vi "ACTION.vi"(8 "error in (no error)":errorcluster, 9 "STEP State":T1, 10 "CORE":refnum<queue>, 11 "Measurement wRelev in":refnum<class "Measurement wRelev.lvclass">) -> (0 "error out":errorcluster, 3 "Measurement wRelev out":refnum<class "Measurement wRelev.lvclass">)   [LabVIEW 2014, in "SeqLoop.lvlib" / "STEP Classes.lvlib" / "Measurement wRelev.lvclass"]
uses:
  Measurement wRelev.lvclass
  TypeDefs/STEP State.ctl
  APIs/Message Queue/Message Cluster.ctl
  Measurement wRelev.lvclass/Measurement wRelev.ctl
  APIs/Message Queue/Enqueue Message (Array).vi
  APIs/Message Queue/Enqueue Message (Single).vi
  APIs/Message Queue/WINFAS 2 Message Queue.lvlib
  SeqLoop.lvlib
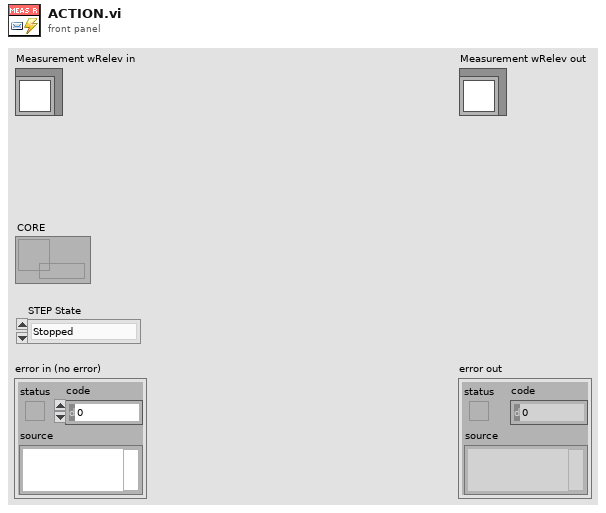
[diagram p1: front panel]
types:
  T1 = typedef "SeqLoop.lvlib/STEP State.ctl" = enum16{"Stopped", "First Call", "Idle...", "Advance OK", "Alarm", "Output Security", "Error"}
  T2 = cluster{"HWSync 1":bool, "HWSync 2":bool, "HWSync 3":bool, "HWSync 4":bool, "HWSync 5":bool}
  T3 = cluster{"HWAsync 1":string, "HWAsync 2":string, "HWAsync 3":string, "HWAsync 4":string, "HWAsync 5":string, "HWAsync 6":string, "HWAsync 7":string, "HWAsync 8":string, "HWAsync 9":string, "HWAsync 10":string}
  T4 = cluster{"format string":string, "Measurement Index":i32[]}
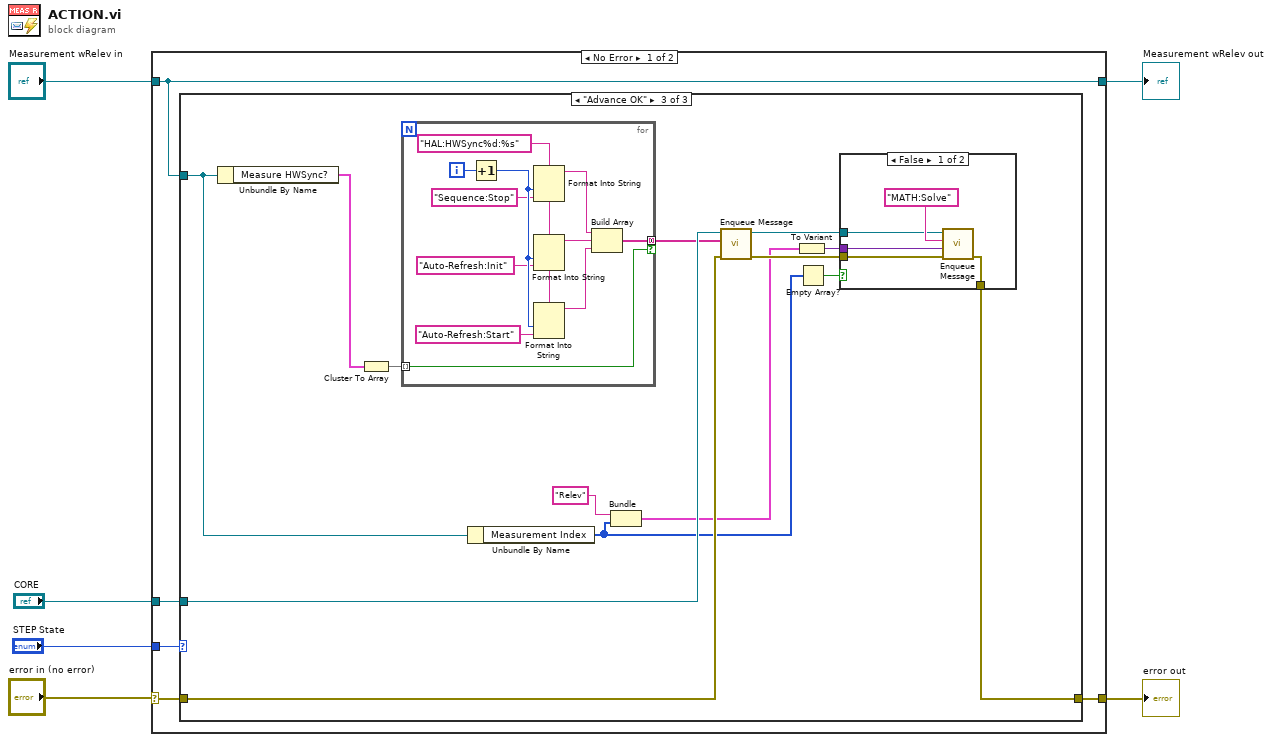
[diagram p0: block diagram]
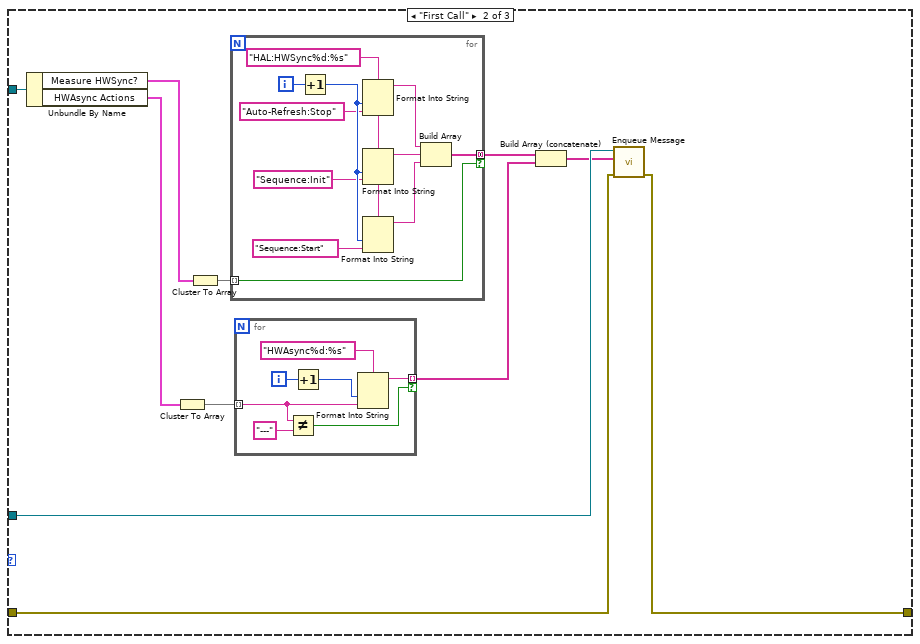
[diagram p3: hidden frame]
diagram:
  n1 = case shown="No Error" "error in (no error)" {
    selector: "error in (no error)" -> [w8 w74]
    tunnel: [w7 w74] -> w3
    tunnel: [w11 w73] -> w5
    tunnel: "Measurement wRelev in" -> [w11 w73]
    tunnel: "CORE" -> [w10 _]
    tunnel: "STEP State" -> [w9 _]
    frame No Error {
      n2 = case shown="\"Advance OK\"" w9 {
        tunnel: w10 -> [_ w16 w53]
        tunnel: w11 -> [_ w22 w50]
        tunnel: w8 -> [w12 w14 w52]
        tunnel: [w12 w13 w42] -> w7
        frame Default {
        }
        frame "First Call" {
          n3 = Unbundle By Name(w22) -> ("Measure HWSync?"=w21:T2, "HWAsync Actions"=w20:T3)
          n4 = Cluster To Array(cluster=w20) -> (array=w19:string[])
          n5 = Cluster To Array(cluster=w21) -> (array=w23:bool[])
          n6 = for {
            tunnel: w23 -> [w31] mode=indexing
            tunnel: [w32] -> w18 mode=concatenating if=w31
            i -> [w41]
            w40 = "HAL:HWSync%d:%s" ("format string")
            n7 = Increment(x=w41) -> (x+1=w39:i32)
            n8 = Format Into String(format string=w40, w39, "Auto-Refresh:Stop" ("format string")) -> (resulting string=w35:string)  [unwired: 2 in, 1 out]
            n9 = Format Into String(format string=w40, w39, "Sequence:Init" ("format string")) -> (resulting string=w34:string)  [unwired: 2 in, 1 out]
            n10 = Format Into String(format string=w40, w39, "Sequence:Start" ("format string")) -> (resulting string=w33:string)  [unwired: 2 in, 1 out]
            n11 = Build Array(w35, w34, w33) -> (w32:string[])
          }
          n12 = for {
            tunnel: w19 -> [w27] mode=indexing
            tunnel: [w25] -> w17 mode=indexing if=w24
            i -> [w29]
            n13 = Not Equal?(x=w27, y="---") -> (x != y?=w24:bool)
            n14 = Increment(x=w29) -> (x+1=w28:i32)
            n15 = Format Into String(format string="HWAsync%d:%s", w28, w27) -> (resulting string=w25:string)  [unwired: 2 in, 1 out]
          }
          n16 = Build Array (concatenate)(w18, w17) -> (w15:string[])
          n17 = call-poly "Enqueue Message.vi"("error in (no error)"=w14, "Message Array"=w15, "Message Queue"=w16) -> ("error out"=w13:errorcluster)  [unwired: 7 in, 1 out]
        }
        frame "Advance OK" {
          n18 = Unbundle By Name(w50) -> ("Measure HWSync?"=w54:T2)
          n19 = Cluster To Array(cluster=w54) -> (array=w55:bool[])
          n20 = for {
            tunnel: w55 -> [w62] mode=indexing
            tunnel: [w63] -> w51 mode=concatenating if=w62
            i -> [w72]
            w71 = "HAL:HWSync%d:%s" ("format string")
            n21 = Increment(x=w72) -> (x+1=w70:i32)
            n22 = Format Into String(format string=w71, w70, "Sequence:Stop" ("format string")) -> (resulting string=w66:string)  [unwired: 2 in, 1 out]
            n23 = Format Into String(format string=w71, w70, "Auto-Refresh:Init" ("format string")) -> (resulting string=w65:string)  [unwired: 2 in, 1 out]
            n24 = Format Into String(format string=w71, w70, "Auto-Refresh:Start" ("format string")) -> (resulting string=w64:string)  [unwired: 2 in, 1 out]
            n25 = Build Array(w66, w65, w64) -> (w63:string[])
          }
          n26 = Unbundle By Name(w50) -> ("Measurement Index"=w43:i32[])
          n27 = Bundle("format string"="Relev", "Measurement Index"=w43) -> (w44:T4)  [unwired: 1 in]
          n28 = call-poly "Enqueue Message.vi"("error in (no error)"=w52, "Message Array"=w51, "Message Queue"=w53) -> ("error out"=w45:errorcluster, "dup Message Queue"=w46:refnum<queue>)  [unwired: 7 in]
          n29 = To Variant(anything=w44) -> (Variant=w48:variant)
          n30 = Empty Array?(array=w43) -> (empty?=w47:bool)
          n31 = case shown="False" w47 {
            tunnel: w45 -> [w60 w61]
            tunnel: [w59 w61] -> w42
            tunnel: w46 -> [w57 _]
            tunnel: w48 -> [w56 _]
            frame False {
              n32 = call-poly "Enqueue Message.vi"("error in (no error)"=w60, "Message Data"=w56, "Message"="MATH:Solve" ("format string"), "Message Queue"=w57) -> ("error out"=w59:errorcluster)  [unwired: 6 in, 1 out]
            }
            frame True {
            }
          }
        }
      }
    }
    frame Error {
    }
  }
  "error out" <- w3
  "Measurement wRelev out" <- w5
